vi "NanoOps New.vi"(8 "error in (no error)":errorcluster, 10 "Toggle time Msecs":dbl, 11 "Cmd":T1) -> (0 "error out":errorcluster={"status"=FALSE, "code"=1073676294, "source"="VISA Read in DoNanoCmd.vi"}, 1 "Return message":string, 2 "Return data":dbl, 3 "Nano out":refnum<visa-resource-name>="COM20")   [LabVIEW 2013]
uses:
  Nano_cmds.ctl
  NanoCmds.ctl
  Test Globals/Global 1.vi
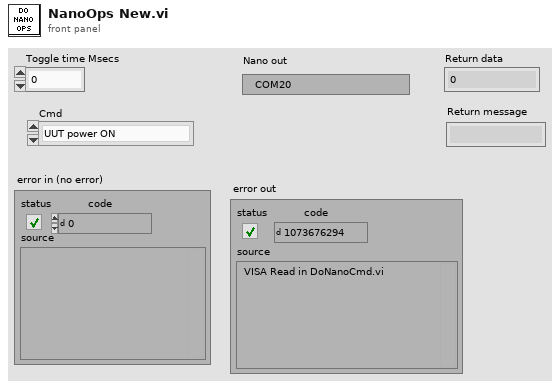
[diagram p1: front panel]
types:
  T1 = typedef "Nano_cmds.ctl" = enum16{"UUT power ON", "UUT power OFF", "Get current draw", "Toggle ON_OFF", "Toggle nReset", "ADC .832vdc", "ADC 0vdc", "Read CTS", "Read nSleep"}
  T2 = typedef "NanoCmds.ctl" = enum16{"Make digital port an output", "Make digital port an input", "Set digital pin high", "Set digital pin low", "Get digital pin state", "Get analog pin voltage", "Get analog pins difference", "Get ohms at analog pin", "Turn on current limit", "Reset Nano device", "Get digital pin state pullup", "Read current", "Initialize", "Power up uut", "Power down uut", "Get uut current draw", "Set ADC volts high", "Set ADC volts low", "Start up uut modem", "Get CTS state", "Get on_nsleep state", "Reset modem", "Get lid state", "Wait for lid closed", "Wait for lid open", "Power up, start, get curr"}
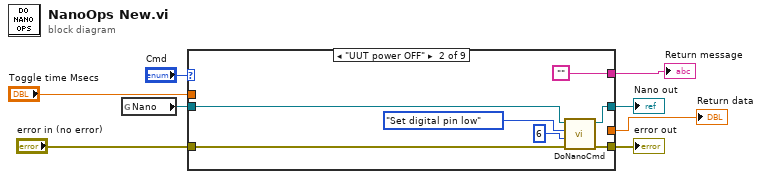
[diagram p0: block diagram]
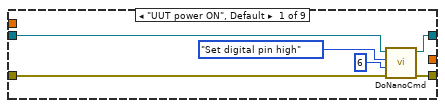
[diagram p2: hidden frame]
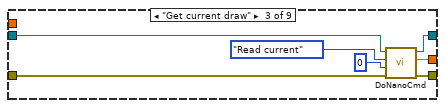
[diagram p3: hidden frame]
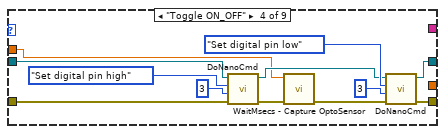
[diagram p4: hidden frame]
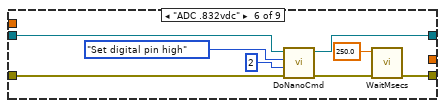
[diagram p6: hidden frame]
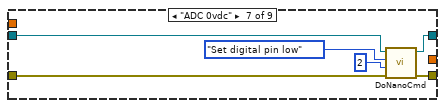
[diagram p7: hidden frame]
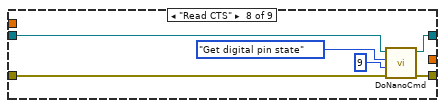
[diagram p8: hidden frame]
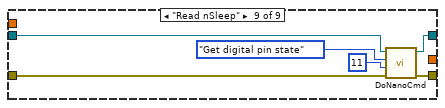
[diagram p9: hidden frame]
diagram:
  n1 = global read "Global 1.vi" "Nano"() -> (w5:refnum<visa-resource-name>)
  n2 = case shown="\"UUT power OFF\"" "Cmd" {
    tunnel: "error in (no error)" -> [w12 w21 w27 w38 w41 w48 w54 w61 w63]
    tunnel: [w10 w20 w26 w33 w41 w44 w52 w60 w64] -> w6
    tunnel: w5 -> [w11 w19 w28 w37 w42 w47 w53 w62 w66]
    tunnel: "Toggle time Msecs" -> [_ _ _ w29 _ _ _ _ _]
    tunnel: [w9 w16 w25 w32 w42 w46 w51 w59 w65] -> w3
    tunnel: [_ _ w22 _ _ _ _ _ _] -> w2
    tunnel: [_ "" _ _ _ _ _ _ _] -> w1
    frame "UUT power ON", Default {
      n3 = call "DoNanoCmd.vi"("error in (no error)"=w12, "Pin 1"=u32 6, "Nano Op"=NanoCmds."Set digital pin high", "VISA resource name"=w11) -> ("error out"=w10:errorcluster, "VISA resource name 2"=w9:refnum<visa-resource-name>)  [unwired: 4 in, 2 out]
    }
    frame "UUT power OFF" {
      n4 = call "DoNanoCmd.vi"("error in (no error)"=w21, "Pin 1"=u32 6, "Nano Op"=NanoCmds."Set digital pin low", "VISA resource name"=w19) -> ("error out"=w20:errorcluster, "VISA resource name 2"=w16:refnum<visa-resource-name>)  [unwired: 4 in, 2 out]
    }
    frame "Get current draw" {
      n5 = call "DoNanoCmd.vi"("error in (no error)"=w27, "Pin 1"=u32 0, "Nano Op"=NanoCmds."Read current", "VISA resource name"=w28) -> ("error out"=w26:errorcluster, "Read Value"=w22:dbl, "VISA resource name 2"=w25:refnum<visa-resource-name>)  [unwired: 4 in, 1 out]
    }
    frame "Toggle ON_OFF" {
      n6 = call "DoNanoCmd.vi"("error in (no error)"=w38, "Pin 1"=u32 3, "Nano Op"=NanoCmds."Set digital pin high", "VISA resource name"=w37) -> ("error out"=w31:errorcluster, "VISA resource name 2"=w34:refnum<visa-resource-name>)  [unwired: 4 in, 2 out]
      n7 = call "WaitMsecs - Capture OptoSensor.vi"("error in (no error)"=w31, "Wait Msecs"=w29) -> ("error out"=w30:errorcluster)  [unwired: 9 in]
      n8 = call "DoNanoCmd.vi"("error in (no error)"=w30, "Pin 1"=u32 3, "Nano Op"=NanoCmds."Set digital pin low", "VISA resource name"=w34) -> ("error out"=w33:errorcluster, "VISA resource name 2"=w32:refnum<visa-resource-name>)  [unwired: 4 in, 2 out]
    }
    frame "Toggle nReset" {
    }
    frame "ADC .832vdc" {
      n9 = call "DoNanoCmd.vi"("error in (no error)"=w48, "Pin 1"=u32 2, "Nano Op"=NanoCmds."Set digital pin high", "VISA resource name"=w47) -> ("error out"=w45:errorcluster, "VISA resource name 2"=w46:refnum<visa-resource-name>)  [unwired: 4 in, 2 out]
      n10 = call "WaitMsecs.vi"("error in (no error)"=w45, "Wait Msecs"=250.0) -> ("error out"=w44:errorcluster)  [unwired: 9 in]
    }
    frame "ADC 0vdc" {
      n11 = call "DoNanoCmd.vi"("error in (no error)"=w54, "Pin 1"=u32 2, "Nano Op"=NanoCmds."Set digital pin low", "VISA resource name"=w53) -> ("error out"=w52:errorcluster, "VISA resource name 2"=w51:refnum<visa-resource-name>)  [unwired: 4 in, 2 out]
    }
    frame "Read CTS" {
      n12 = call "DoNanoCmd.vi"("error in (no error)"=w61, "Pin 1"=u32 9, "Nano Op"=NanoCmds."Get digital pin state", "VISA resource name"=w62) -> ("error out"=w60:errorcluster, "VISA resource name 2"=w59:refnum<visa-resource-name>)  [unwired: 4 in, 2 out]
    }
    frame "Read nSleep" {
      n13 = call "DoNanoCmd.vi"("error in (no error)"=w63, "Pin 1"=u32 11, "Nano Op"=NanoCmds."Get digital pin state", "VISA resource name"=w66) -> ("error out"=w64:errorcluster, "VISA resource name 2"=w65:refnum<visa-resource-name>)  [unwired: 4 in, 2 out]
    }
  }
  "error out" <- w6
  "Nano out" <- w3
  "Return data" <- w2
  "Return message" <- w1
